vi "hmi_simulacionRK4.vi"() -> ()   [LabVIEW 2017]
uses:
  Control 6.ctl
  <vilib>/Platform/TimedLoop/XDataNode/timing_clust.ctl
  <vilib>/Platform/TimedLoop/XDataNode/nitl_modes.ctl
  <vilib>/Platform/TimedLoop/XDataNode/wakeup.ctl
  <vilib>/platform/TimedLoop/XDataNode/XDataNode.xnode
  <vilib>/Platform/TimedLoop/XDataNode/XDNodeRunTimeDep.lvlib
panel:
  in  "Tab Control":enum32{"HMI", "Monitorizacion de flujo"}(tab)
  in  "Presion de salida":dbl caption="MPa"
  in  "Presion de entrada":dbl caption="MPa"
  out "PT-002":dbl caption="MPa"
  out "PT-001":dbl caption="MPa"
  in  "Flujo de entrada":dbl caption="L/min"
  in  "Flujo de salida":dbl caption="L/min"
  out "Boolean 2":bool
  out "FUGA 1":bool
  out "FUGA 2":bool
  out "Boolean":bool
  in  "stop 2":bool
  in  "BOMBA ON/OFF":bool
  out "FT1":bool(c317)
  out "TANQUE\n FLUIDO:AGUA":dbl(slide) scale=0.0..100.0
  in  "valvula 1":bool
  in  "valvula 2":bool
  in  "ts":dbl caption="ms"
  out "TEE 02":bool
  out "TUBERIA 1IN TRAMO 02":bool(c317)
  out "TEE1":bool
  out "Multi-Segment Pipe 2":T1
  out "Multi-Segment Pipe 3":bool(c317)
  out "BOMBA  PERIFERICA1/2 HP":bool
  out "codo90":bool
  out "Multi-Segment Pipe 4":bool(c317)
  out "FT2":bool(c317)
  in  "u1":dbl
  in  "u2":dbl
  in  "tiempo de simulacion":i64=8
  out "FT -001":dbl caption="L/min"
  out "FT-002":dbl caption="L/min"
  out "SENSOR FLUJO 4":bool
  out "SENSOR FLUJO 5":bool
  out "Tiempo":dbl caption="s"
  out "XY Graph":cluster{dbl[], dbl[]}(graph)
  in  "Guardar  a Excel":bool
  out "Flujo de entrada y salida":cluster{dbl[], dbl[]}[](graph)
  in  "stop":bool
  # "PVC  1\" FLUJO: AGUA"
  # "PVC  1/2\" FLUJO: AGUA"
  # "FUGA 1"
  # "2.5 m"
  # "PVC  1/2\" FLUJO: AGUA"
  # "FUGA 2"
  # "PVC  1\" FLUJO: AGUA"
  # "9 m"
  # "Grafica de flujo en sensores YF-S201"
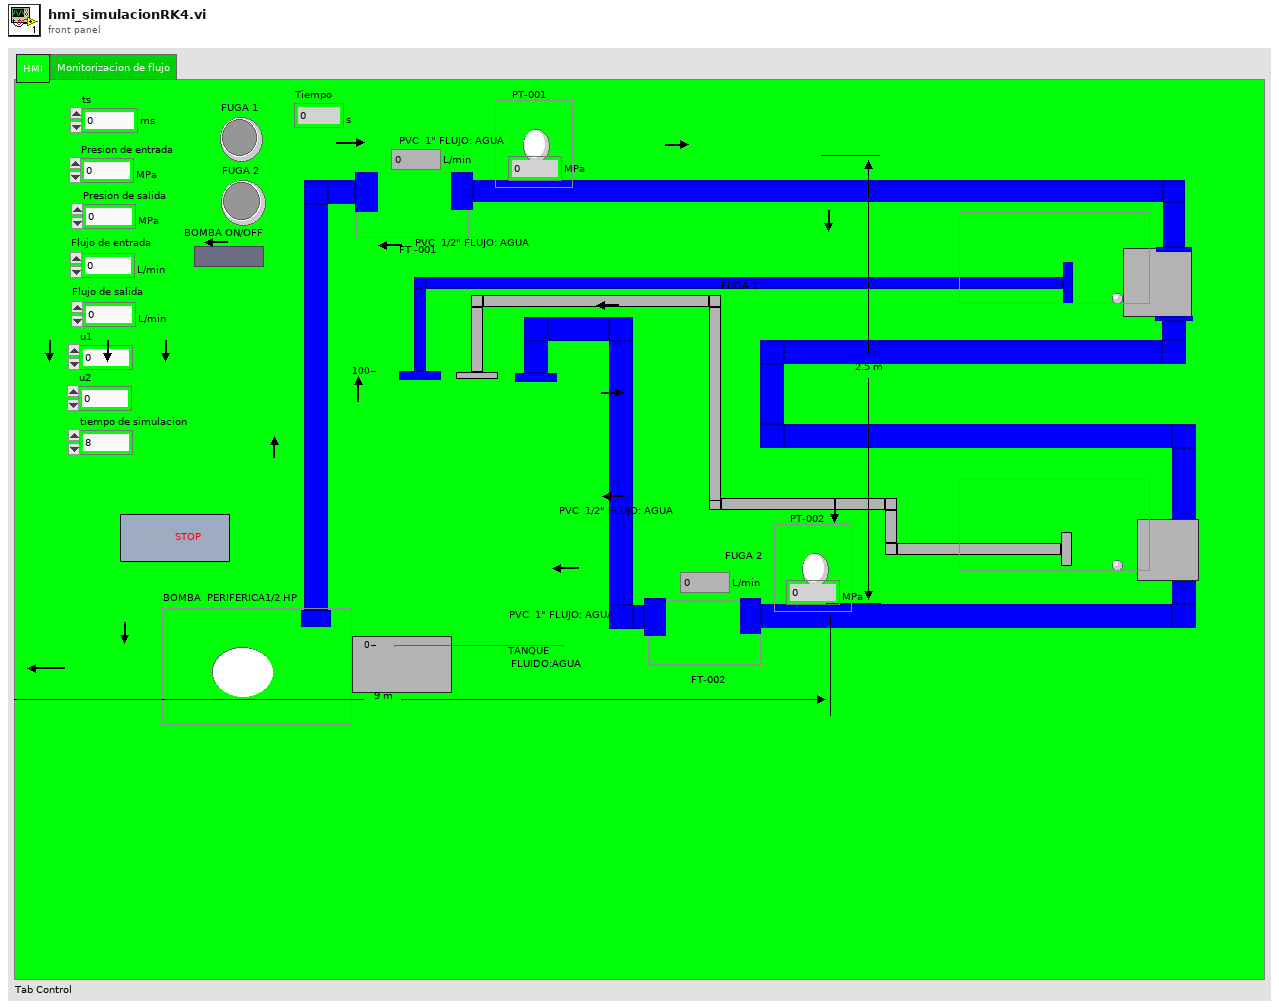
[diagram p1: front panel]
types:
  T1 = typedef "Control 6.ctl" = bool
  T2 = typedef "XDNodeRunTimeDep.lvlib/timing_clust.ctl" = cluster{"Expected End [f-1]":u64, "Actual End [f-1]":u64, "Finished Late? [f-1]":bool, "Expected End [i-1]":u64, "Actual End [i-1]":u64, "Finished Late? [i-1]":bool, "Expected Start [i]":u64, "Actual Start [i]":u64, "Expected Start [f]":u64, "Actual Start [f]":u64, "Source Name":string, "Structure Name":string, "Period":i64, "Deadline":i64, "Offset":i64, "Start":i64, "Priority":i32, "Timeout":i32, "Mode":T3, "Wakeup Reason":T4, "Error":errorcluster, "Source Type":string, "Secondary Source Type":string, "Global End Time":u64, "Global Start Time":u64, "Frame Duration":u64, "Iteration Duration":u64, "Assigned CPU":i32, "I/O Scan Engine Mode":u32}
  T3 = typedef "XDNodeRunTimeDep.lvlib/nitl_modes.ctl" = enum32{"No Change", "Process missed periods, maintain original phase", "Discard missed periods, maintain original phase", "Process missed periods, ignore original phase", "Discard missed periods, ignore original phase"}
  T4 = typedef "XDNodeRunTimeDep.lvlib/wakeup.ctl" = enum32{"Normal", "Aborted", "Asynchronous wakeup", "Timing source error", "Timed loop error", "Timeout"}
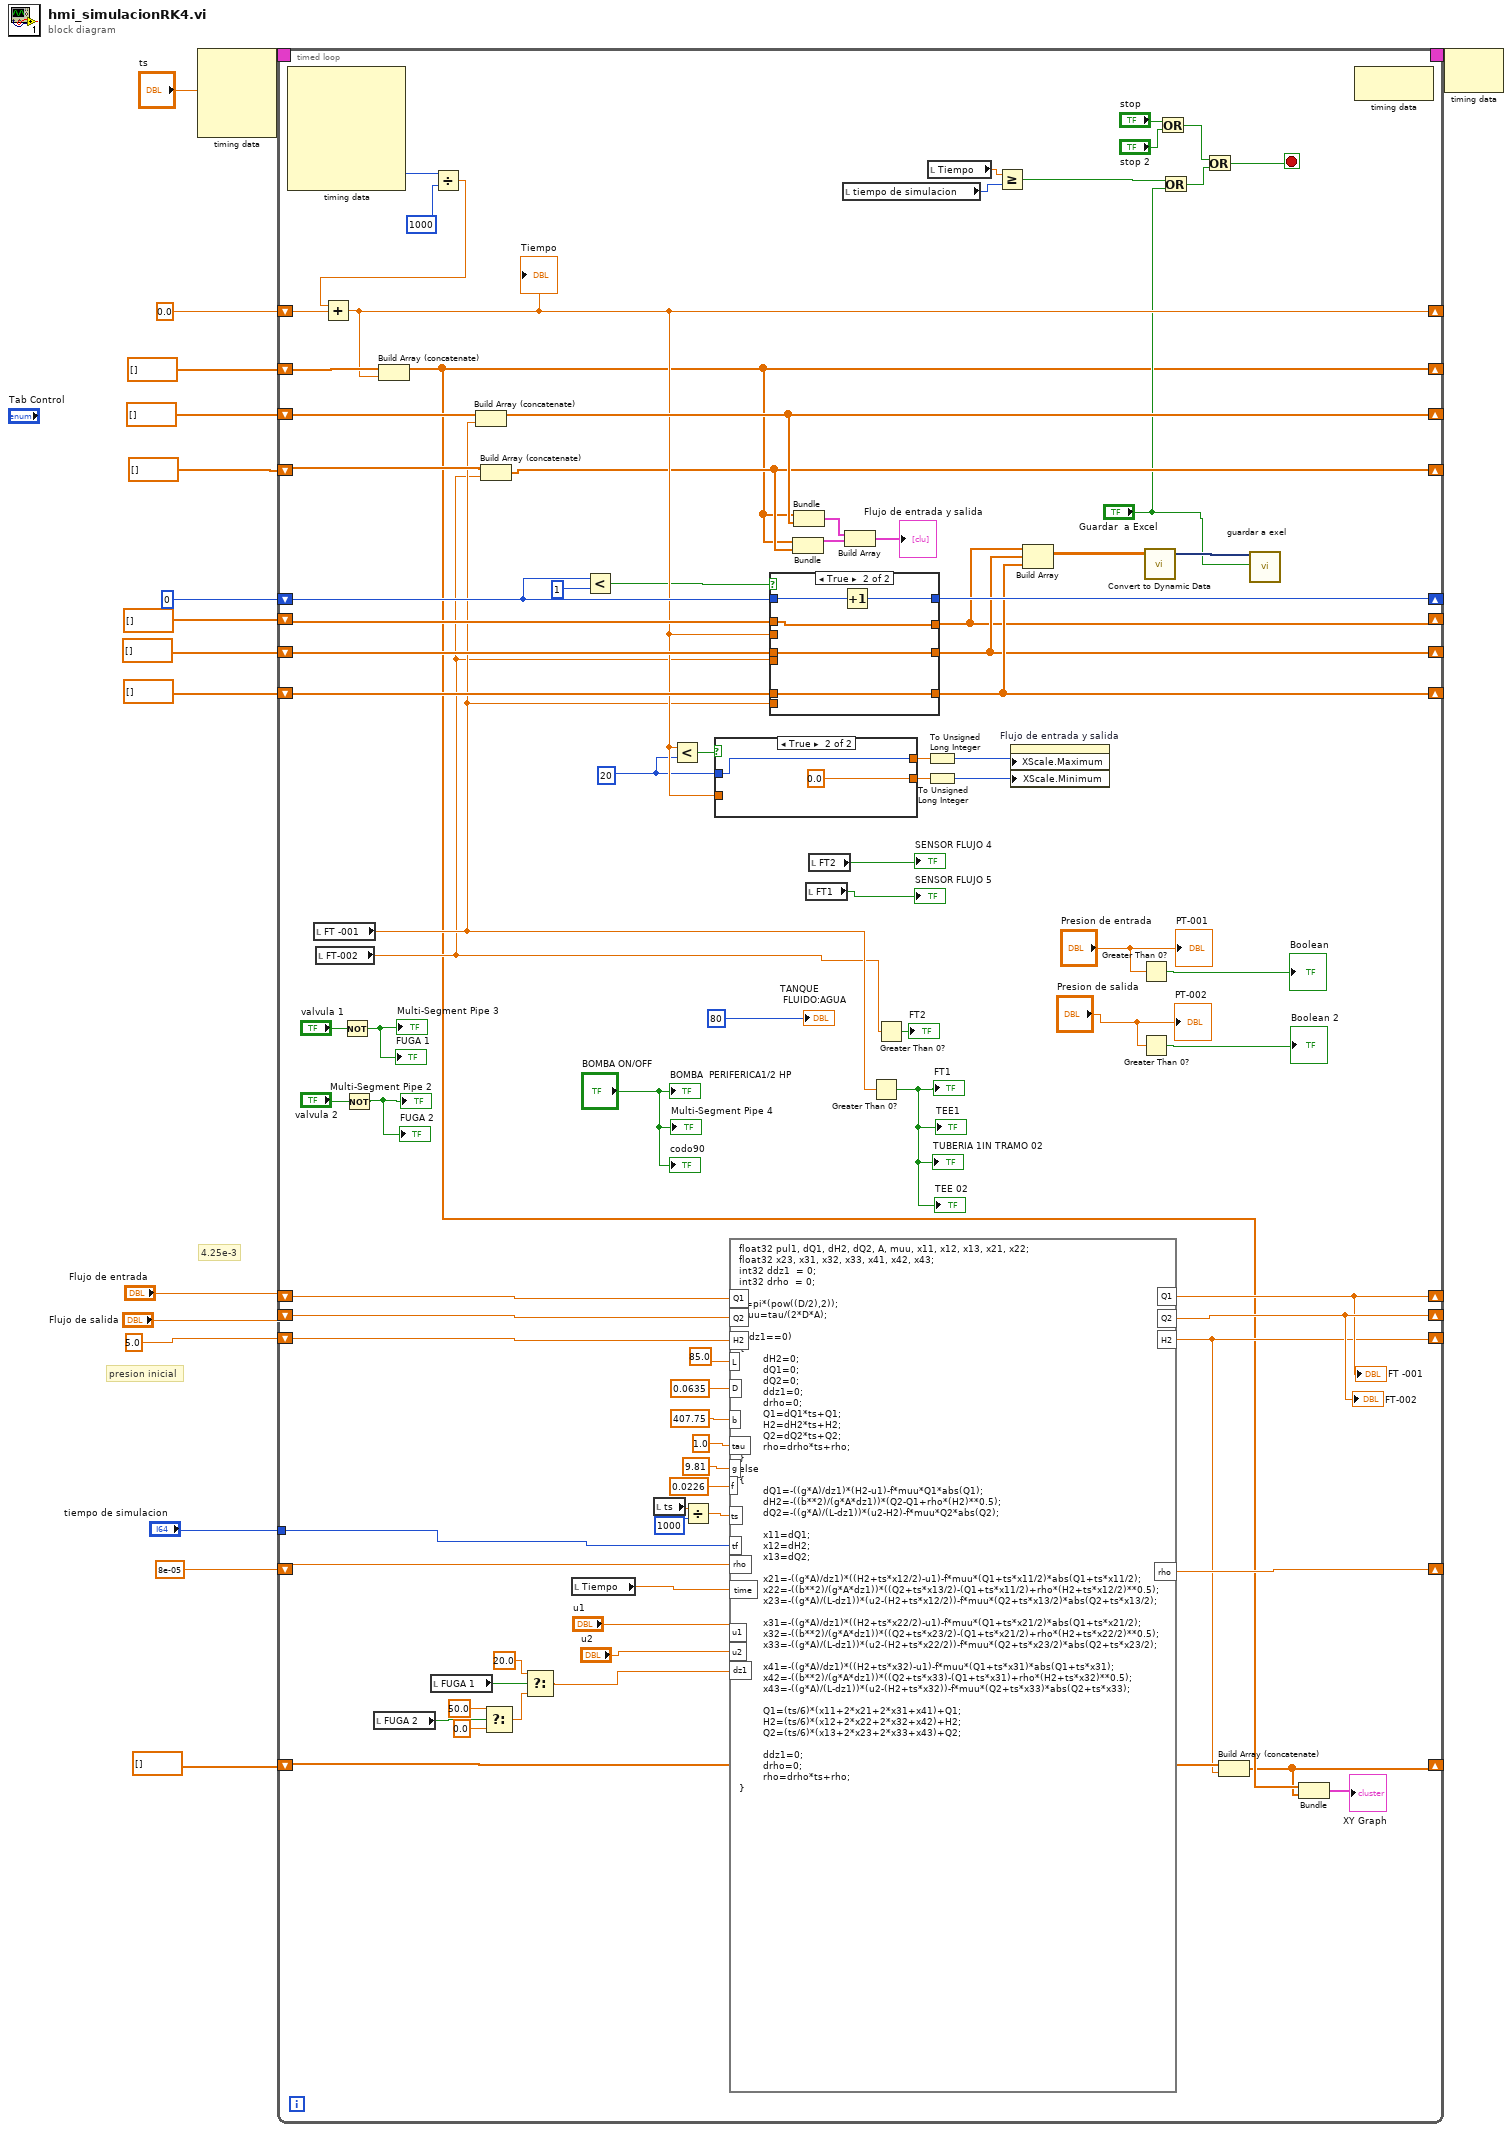
[diagram p0: block diagram]
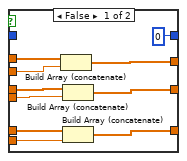
[diagram p2: hidden frame]
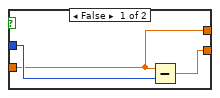
[diagram p3: hidden frame]
diagram:
  # "4.25e-3"
  # "presion inicial"
  n1 = node-c288("ts") -> (w9:T2)  [unwired: 3 in]
  n2 = timed-loop {
    shift-right: [w22] -> _
    shift-left: dbl[] [] -> [w104]
    shift-right: [w87] -> _
    shift-left: 0.0 -> [w105]
    shift-right: [w97] -> _
    shift-left: dbl[] [] -> [w102]
    shift-right: [w78] -> _
    shift-left: dbl[] [] -> [w103]
    shift-right: [w93] -> _
    shift-left: 0 -> [w94]
    shift-right: [w88] -> _
    shift-left: dbl[] [] -> [w91]
    shift-right: [w89] -> _
    shift-left: dbl[] [] -> [w90]
    shift-right: [w86] -> _
    shift-left: dbl[] [] -> [w92]
    timing: w9 -> [_]
    timing-out: [_] -> w8
    shift-right: [w38] -> _
    shift-left: "Flujo de salida" -> [w40]
    shift-right: [w37] -> _
    shift-left: "Flujo de entrada" -> [w39]
    shift-right: [w33] -> _
    shift-left: 5.0 -> [w52]
    shift-right: [w48] -> _
    shift-left: 8e-05 ("input variable") -> [w49]
    tunnel: "tiempo de simulacion" -> [w43]
    shift-right: [w21] -> _
    shift-left: dbl[] [] -> [w34]
    stop <- w96 stop-if-true
    w18 = i16 20 ("Rango de grafica")
    n3 = node-c288() -> (w64:i64)  [unwired: 1 in, 6 out]
    n4 = local read "FT -001"() -> (w36:dbl)
    n5 = local read "FT-002"() -> (w35:dbl)
    n6 = Not(x="valvula 1") -> (.not. x?=→"Multi-Segment Pipe 3" →"FUGA 1":bool)
    n7 = Not(x="valvula 2") -> (.not. x?=→"Multi-Segment Pipe 2" →"FUGA 2":bool)
    n8 = local read "FUGA 2"() -> (w29:bool)
    n9 = local read "FUGA 1"() -> (w31:bool)
    n10 = Divide(x=w64, y=i64 1000) -> (x/y=w63:dbl)
    n11 = Add(x=w63, y=w105) -> (x+y=w87:dbl)
    "Tiempo" <- w87
    n12 = Build Array (concatenate)(w104, w87) -> (w22:dbl[])
    n13 = Build Array (concatenate)(w102, w36) -> (w97:dbl[])
    n14 = Build Array (concatenate)(w103, w35) -> (w78:dbl[])
    n15 = Select(t=50.0, s=w29, f=0.0) -> (s? t:f=w28:dbl)
    n16 = Select(t=20.0, s=w31, f=w28) -> (s? t:f=w32:dbl)
    n17 = local read "Tiempo"() -> (w41:dbl)
    n18 = Less?(x=w94, y=u32 1) -> (x < y?=w79:bool)
    n19 = local read "ts"() -> (w54:dbl)
    n20 = Less?(x=w87, y=w18) -> (x < y?=w99:bool)
    n21 = Divide(x=w54, y=1000) -> (x/y=w53:dbl)
    n22 = case shown="True" w99 {
      tunnel: w18 -> [w125 w127]
      tunnel: [w124 w127] -> w83
      tunnel: [w126 0.0] -> w81
      tunnel: w87 -> [w124 _]
      frame False {
        n23 = Subtract(x=w124, y=w125) -> (x-y=w126:dbl)
      }
      frame True {
      }
    }
    n24 = formula code="float32 pul1, dQ1, dH2, dQ2, A, muu, x11, x12, x13, x21, x22;\nfloat32 x23, x31, x32, x33, x41, x42, x43;\nint32 ddz1  = 0;\nint32 drho  = 0;\n\nA=pi*(pow((D/2),2));\nmuu=tau/(2*D*A);\n\nif(dz1==0)\n{\n        dH2=0;\n        dQ1=0;\n        dQ2=0;\n        ddz1=0;\n        drho=0;\n        Q1=dQ1*ts+Q1;\n        H2=dH2*ts+H2;    \n        Q2=dQ2*ts+Q2;\n        rho=drho*ts+rho;\n}\nelse \n{\n        dQ1=-((g*A)/dz1)*(H2-u1)-f*muu*Q1*abs(Q1);\n        dH2=-((b**2)/(g*A*dz1))*(Q2-Q1+rho*(H2)**0.5);\n        dQ2=-((g*A)/(L-dz1))*(u2-H2)-f*muu*Q2*abs(Q2);\n        \n        x11=dQ1;\n        x12=dH2;\n        x13=dQ2;\n        \n        x21=-((g*A)/dz1)*((H2+ts*x12/2)-u1)-f*muu*(Q1+ts*x11/2)*abs(Q1+ts*x11/2);\n        x22=-((b**2)/(g*A*dz1))*((Q2+ts*x13/2)-(Q1+ts*x11/2)+rho*(H2+ts*x12/2)**0.5);\n        x23=-((g*A)/(L-dz1))*(u2-(H2+ts*x12/2))-f*muu*(Q2+ts*x13/2)*abs(Q2+ts*x13/2);\n        \n        x31=-((g*A)/dz1)*((H2+ts*x22/2)-u1)-f*muu*(Q1+ts*x21/2)*abs(Q1+ts*x21/2);\n        x32=-((b**2)/(g*A*dz1))*((Q2+ts*x23/2)-(Q1+ts*x21/2)+rho*(H2+ts*x22/2)**0.5);\n        x33=-((g*A)/(L-dz1))*(u2-(H2+ts*x22/2))-f*muu*(Q2+ts*x23/2)*abs(Q2+ts*x23/2);\n        \n        x41=-((g*A)/dz1)*((H2+ts*x32)-u1)-f*muu*(Q1+ts*x31)*abs(Q1+ts*x31);\n        x42=-((b**2)/(g*A*dz1))*((Q2+ts*x33)-(Q1+ts*x31)+rho*(H2+ts*x32)**0.5);\n        x43=-((g*A)/(L-dz1))*(u2-(H2+ts*x32))-f*muu*(Q2+ts*x33)*abs(Q2+ts*x33);\n        \n        Q1=(ts/6)*(x11+2*x21+2*x31+x41)+Q1;\n        H2=(ts/6)*(x12+2*x22+2*x32+x42)+H2;\n        Q2=(ts/6)*(x13+2*x23+2*x33+x43)+Q2;\n        \n        ddz1=0;\n        drho=0;\n        rho=drho*ts+rho;\n}"("L"=85.0, "D"=0.0635, "b"=407.75 ("input variable"), "tau"=1.0 ("input variable"), "g"=9.81 ("input variable"), "Q1"=w39, "Q2"=w40, "f"=0.0226 ("input variable"), "ts"=w53, "tf"=w43, "rho"=w49, "H2"=w52, "time"=w41, "u1"="u1", "u2"="u2", "dz1"=w32) -> ("rho"=w48:dbl, "Q1"=w37:dbl, "Q2"=w38:dbl, "H2"=w33:dbl)
    "FT -001" <- w37
    "FT-002" <- w38
    n25 = case shown="True" w79 {
      tunnel: w94 -> [_ w123]
      tunnel: [u32 0 w122] -> w93
      tunnel: w92 -> [w117 w119]
      tunnel: w35 -> [w115 _]
      tunnel: [w118 w121] -> w88
      tunnel: w91 -> [w116 w121]
      tunnel: w36 -> [w113 _]
      tunnel: w90 -> [w114 w120]
      tunnel: [w112 w120] -> w89
      tunnel: [w111 w119] -> w86
      tunnel: w87 -> [w110 _]
      frame False {
        n26 = Build Array (concatenate)(w117, w110) -> (w111:dbl[])
        n27 = Build Array (concatenate)(w116, w115) -> (w118:dbl[])
        n28 = Build Array (concatenate)(w114, w113) -> (w112:dbl[])
      }
      frame True {
        n29 = Increment(x=w123) -> (x+1=w122:u32)
      }
    }
    n30 = Bundle(w22, w78) -> (w100:cluster{dbl[], dbl[]})  [unwired: 1 in]
    n31 = Bundle(w22, w97) -> (w101:cluster{dbl[], dbl[]})  [unwired: 1 in]
    n32 = local read "FT1"() -> (→"SENSOR FLUJO 5":bool)
    n33 = local read "FT2"() -> (→"SENSOR FLUJO 4":bool)
    n34 = local read "tiempo de simulacion"() -> (w42:i64)
    n35 = Build Array(w101, w100) -> (→"Flujo de entrada y salida":cluster{dbl[], dbl[]}[])
    n36 = Greater Than 0?(x=w36) -> (x > 0?=→"TUBERIA 1IN TRAMO 02" →"TEE1" →"TEE 02" →"FT1":bool)
    n37 = Greater Than 0?(x=w35) -> (x > 0?=→"FT2":bool)
    n38 = To Unsigned Long Integer(number=w83) -> (unsigned 32bit integer=w82:u32)
    n39 = To Unsigned Long Integer(number=w81) -> (unsigned 32bit integer=w80:u32)
    n40 = local read "Tiempo"() -> (w45:dbl)
    n41 = Greater Or Equal?(x=w45, y=w42) -> (x >= y?=w44:bool)
    n42 = property on="Flujo de entrada y salida" class="XYGraph (strict)"("XScale.Maximum"=w82, "XScale.Minimum"=w80) -> ()  [unwired: 2 in, 2 out]
    n43 = Build Array(w86, w88, w89) -> (w84:dbl[][])
    n44 = Greater Than 0?(x="Presion de entrada") -> (x > 0?=→"Boolean":bool)
    n45 = Greater Than 0?(x="Presion de salida") -> (x > 0?=→"Boolean 2":bool)
    n46 = call "Convert to Dynamic Data"("2D Array"=w84) -> ("Dynamic Data Type"=w85:dynamicdata)  [unwired: 3 in]
    n47 = Or(x="stop", y="stop 2") -> (x .or. y?=w72:bool)
    n48 = Or(x=w44, y="Guardar  a Excel") -> (x .or. y?=w46:bool)
    n49 = Or(x=w72, y=w46) -> (x .or. y?=w96:bool)
    n50 = Build Array (concatenate)(w34, w33) -> (w21:dbl[])
    n51 = call "guardar a exel"("Signals"=w85, "Enable"="Guardar  a Excel") -> ()  [unwired: 15 in, 3 out]
    n52 = Bundle(w22, w21) -> (→"XY Graph":cluster{dbl[], dbl[]})  [unwired: 1 in]
    n53 = node-c288() -> ()  [unwired: 1 in, 1 out]
    "TANQUE\n FLUIDO:AGUA" <- 80
    "BOMBA  PERIFERICA1/2 HP" <- "BOMBA ON/OFF"
    "codo90" <- "BOMBA ON/OFF"
    "Multi-Segment Pipe 4" <- "BOMBA ON/OFF"
    "PT-001" <- "Presion de entrada"
    "PT-002" <- "Presion de salida"
  }
  n54 = node-c288(w8) -> ()  [unwired: 1 out]
